vi "rm.server.visualize.vi"(8 "error in (no error)":errorcluster, 11 "Item Ref in":T1 format="%.0x") -> (0 "error out":errorcluster, 3 "Item Ref out":T1 format="%.0x")   [LabVIEW 2016, in "RM.Server.lvlib"]
uses:
  RM.Server.lvlib
  <vilib>/NI Veristand/Custom Device API/Custom Device Item Ref.ctl
  viz_entry.ctl
  viz_type.ctl
  viz_show.ctl
  viz_state.ctl
  <vilib>/NI Veristand/Custom Device Tools/Custom Device Utility Library/Custom Device Utility Library.lvlib
  <vilib>/NI Veristand/Custom Device API/Custom Device API.lvlib
panel:
  in  "Collapse Sidebar":bool
  in  "Collapse Sort Options":bool
  in  "Sort By...":T2 items=["RIO device", "resource", "input type", "datatype", "reserver"]
  in  "Collapse Filter Options":bool
  in  "Show":T3
  in  "Display":i32(listbox)
  out "selected values":bool[](array[boolean])
  in  "table":i32(listbox)
  out "resource entries":T4[](array[typedef]) {"FPGA CD Ref" format="%.0x"; "reserver" format="%.0x"}
  # "Options"
  # "Sort"
  # "Filter"
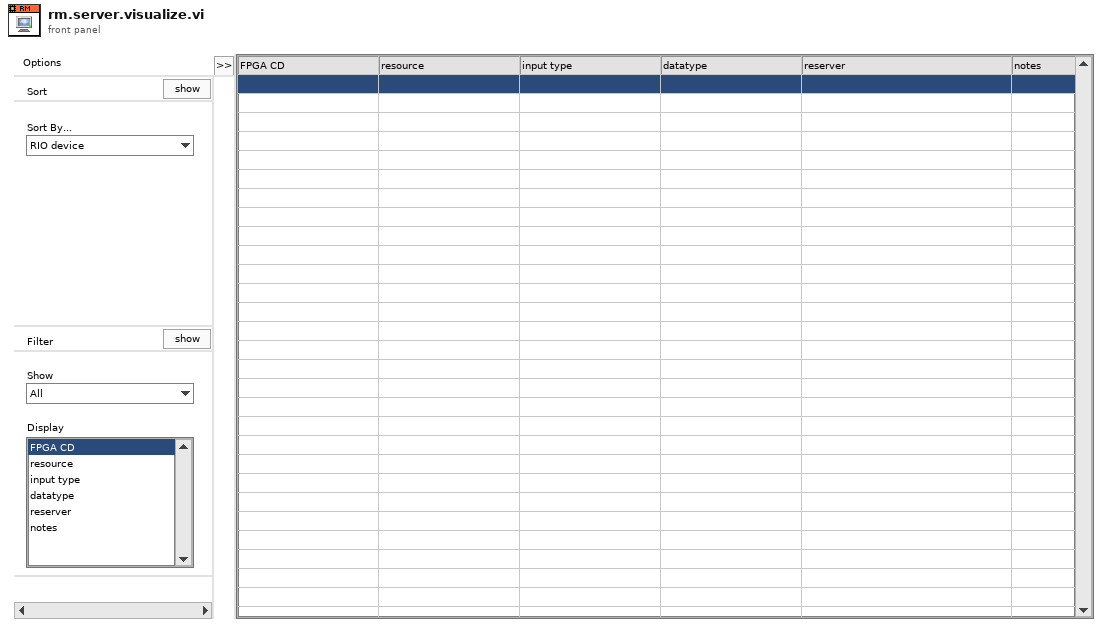
[diagram p1: front panel]
types:
  T1 = typedef "Custom Device API.lvlib/Custom Device Item Ref.ctl" = u64
  T2 = typedef "RM.Server.lvlib/viz_type.ctl" = u16
  T3 = typedef "RM.Server.lvlib/viz_show.ctl" = enum16{"All", "Mapped", "Unmapped"}
  T4 = typedef "RM.Server.lvlib/viz_entry.ctl" = cluster{"FPGA CD Ref":T1, "resource name":string, "input type":string, "datatype":string, "reserver":T1, "notes":string}
  T5 = typedef "RM.Server.lvlib/viz_state.ctl" = enum16{"shutdown"}
  T6 = typedef "RM.Server.lvlib/viz_command.ctl" = cluster{"state":T5, "data":variant}
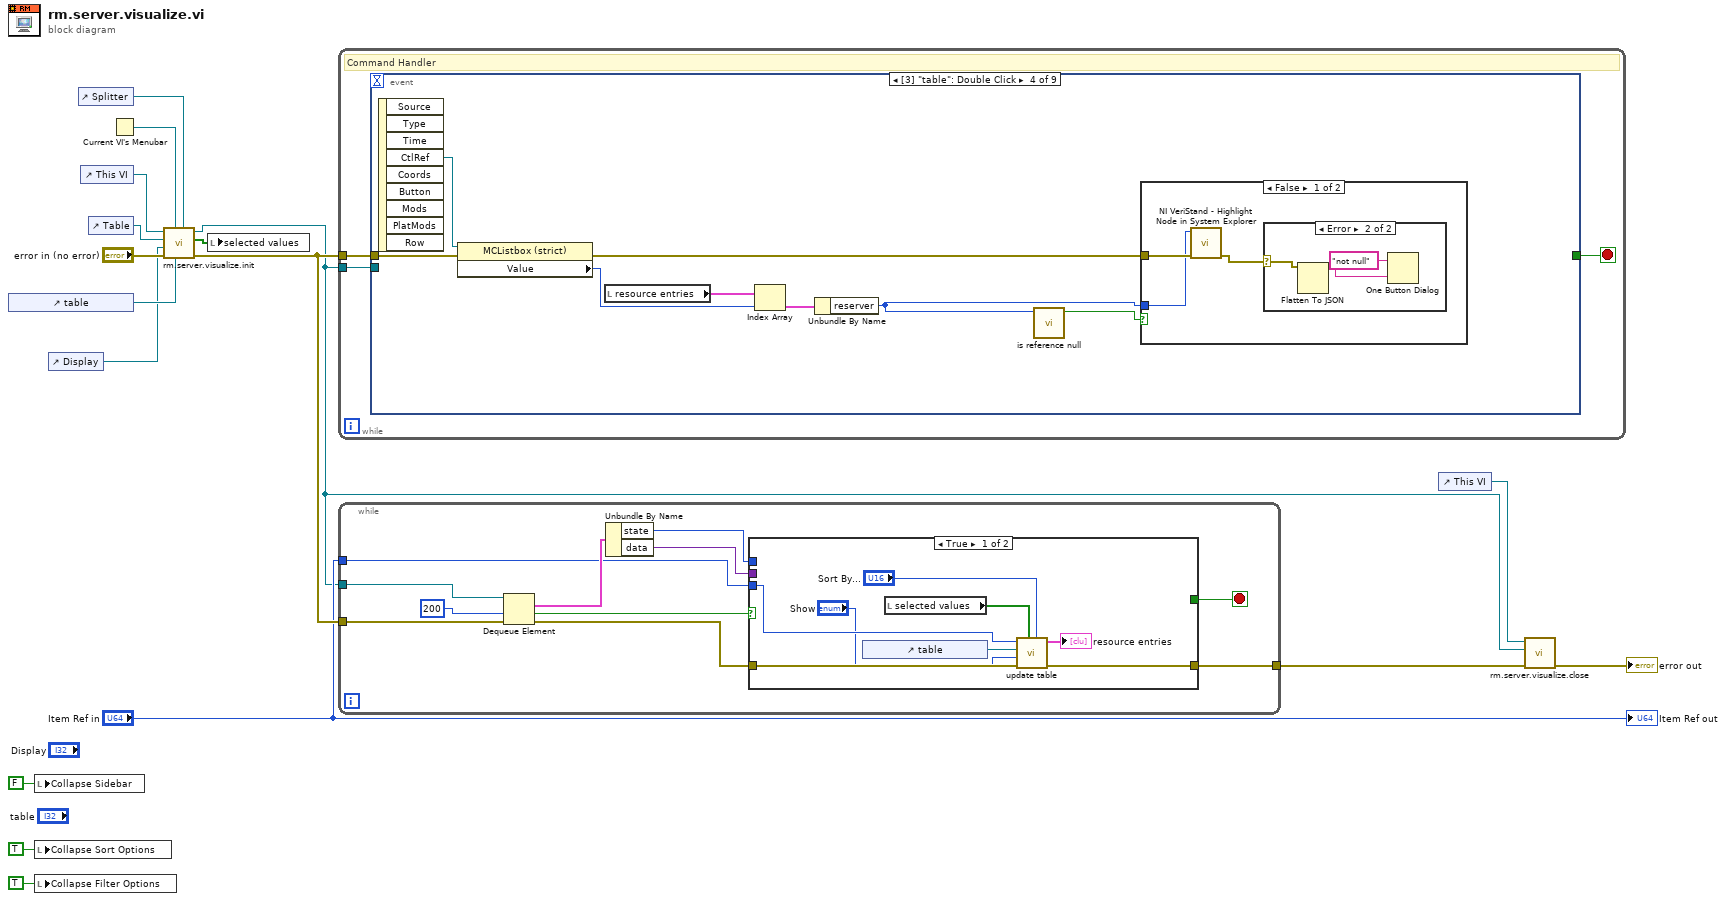
[diagram p0: block diagram]
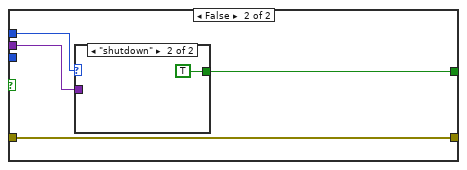
[diagram p2: hidden frame]
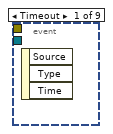
[diagram p4: hidden frame]
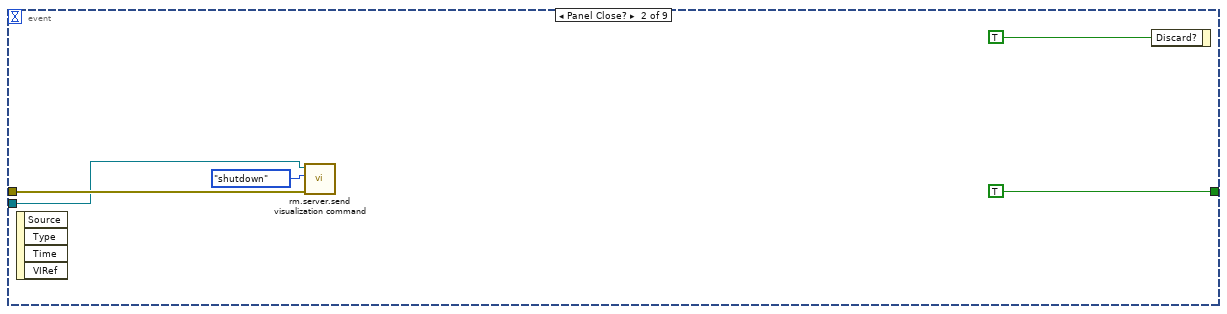
[diagram p5: hidden frame]
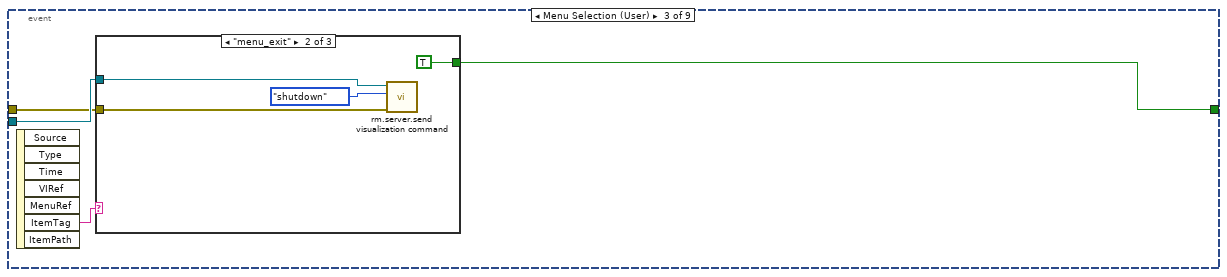
[diagram p6: hidden frame]
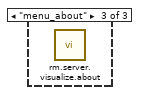
[diagram p8: hidden frame]
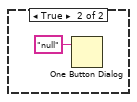
[diagram p10: hidden frame]
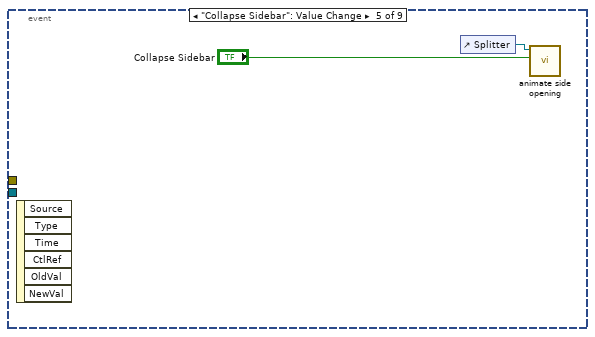
[diagram p11: hidden frame]
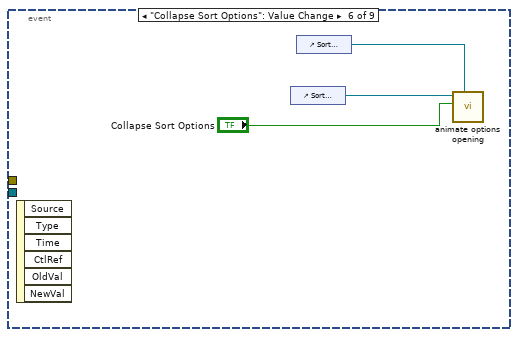
[diagram p12: hidden frame]
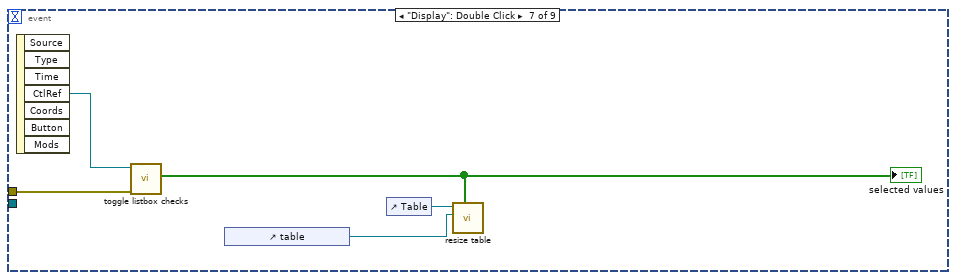
[diagram p13: hidden frame]
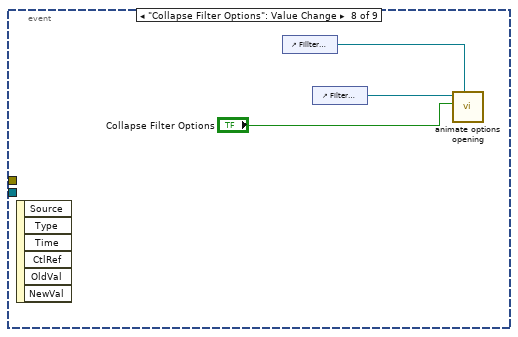
[diagram p14: hidden frame]
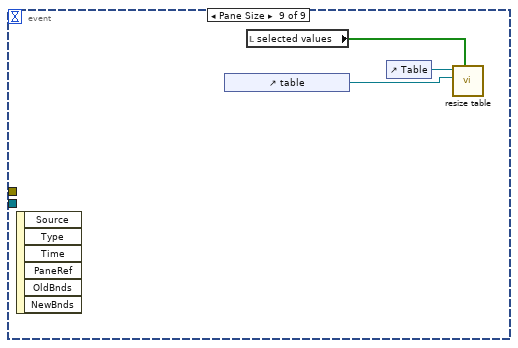
[diagram p15: hidden frame]
diagram:
  n1 = control-ref of="table"() -> (w4:refnum<vi>)
  n2 = local write "Collapse Sidebar"(FALSE ("Collapse Sidebar")) -> ()
  n3 = local write "Collapse Sort Options"(TRUE ("Collapse Sort Options")) -> ()
  n4 = local write "Collapse Filter Options"(TRUE ("Collapse Sort Options")) -> ()
  n5 = control-ref of="Display"() -> (w1:refnum<vi>)
  n6 = control-ref of="Splitter"() -> (w8:refnum<vi>)
  n7 = control-ref of="This VI"() -> (w14:refnum<vi>)
  n8 = control-ref of="Table"() -> (w3:refnum<vi>)
  n9 = Current VI's Menubar() -> (w9:refnum<k9>)
  n10 = call "rm.server.visualize.init.vi"("Splitter"=w8, "MCLB Reference"=w4, "menu reference in"=w9, "error in (no error)"="error in (no error)", "display"=w1, "Table Pane in"=w3, "VI in"=w14) -> ("error out"=w16:errorcluster, "selected values"=w2:bool[], "Queue out"=w10:refnum<queue>)  [unwired: 2 in]
  n11 = local write "selected values"(w2) -> ()
  n12 = while {
    tunnel: w10 -> [w19]
    tunnel: w16 -> [w18]
    stop <- w20 stop-if-true
    # "Command Handler"
    n13 = event shown="[3] \"table\": Double Click" {
      selector: _ -> [_ _ _ _ _ _ _ _ _]
      dyn-events: _ -> [_ _ _ _ _ _ _ _ _]
      timeout: _ -> [_ _ _ _ _ _ _ _ _]
      tunnel: [_ TRUE w28 _ _ _ _ _ _] -> w20
      tunnel: w19 -> [_ w21 w27 _ _ _ _ _ _]
      tunnel: w18 -> [_ w22 w26 w40 _ _ w57 _ _]
      event Timeout {
        n14 = event-data() -> ()  [unwired: 1 in, 3 out]
      }
      event Panel Close? {
        n15 = event-data() -> ()  [unwired: 1 in, 4 out]
        n16 = call "rm.server.send visualization command.vi"("error in (no error)"=w22, "state"=viz_state."shutdown" ("viz_state"), "Queue in"=w21) -> ()  [unwired: 8 in, 1 out]
        n17 = event-data("Discard?"=TRUE ("SilentShutdown")) -> ()  [unwired: 1 in, 1 out]
      }
      event Menu Selection (User) {
        n18 = event-data() -> ("ItemTag"=w29:string)  [unwired: 1 in, 6 out]
        n19 = case shown="\"menu_exit\"" w29 {
          tunnel: [_ TRUE _] -> w28
          tunnel: w27 -> [_ w32 _]
          tunnel: w26 -> [_ w30 _]
          frame Default {
          }
          frame "menu_exit" {
            n20 = call "rm.server.send visualization command.vi"("error in (no error)"=w30, "state"=viz_state."shutdown" ("viz_state"), "Queue in"=w32) -> ()  [unwired: 8 in, 1 out]
          }
          frame "menu_about" {
            n21 = call "rm.server.visualize.about.vi"() -> ()  [unwired: 12 in]
          }
        }
      }
      event "table": Double Click {
        n22 = event-data() -> ("CtlRef"=w41:refnum<vi>)  [unwired: 1 in, 8 out]
        n23 = property class="MCListbox (strict)"(reference=w41, error in=w40) -> (error out=w38:errorcluster, "Value"=w39:i32)  [unwired: 1 out]
        n24 = local read "resource entries"() -> (w37:T4[])
        n25 = Index Array(array=w37, index=w39) -> (element=w36:T4)
        n26 = Unbundle By Name(w36) -> ("reserver"=w35:T1)
        n27 = call "is reference null.vi"("reserver"=w35) -> ("Boolean"=w34:bool)  [unwired: 10 in]
        n28 = case shown="False" w34 {
          tunnel: w38 -> [w44 _]
          tunnel: w35 -> [w43 _]
          frame False {
            n29 = call <vilib>:"NI VeriStand - Highlight Node in System Explorer.vi"("error in (no error)"=w44, "Item Ref in"=w43) -> ("error out"=w42:errorcluster)  [unwired: 8 in, 1 out]
            n30 = case shown="Error" w42 {
              selector: w42 -> [_ w46]
              frame No Error {
              }
              frame Error {
                n31 = Flatten To JSON(anything=w46) -> (JSON string=w45:string)  [unwired: 2 in, 1 out]
                n32 = One Button Dialog(message="not null", button name ("OK")=w45) -> ()  [unwired: 1 out]
              }
            }
          }
          frame True {
            n33 = One Button Dialog(message="null") -> ()  [unwired: 1 in, 1 out]
          }
        }
      }
      event "Collapse Sidebar": Value Change {
        n34 = event-data() -> ()  [unwired: 1 in, 6 out]
        n35 = control-ref of="Splitter"() -> (w50:refnum<vi>)
        n36 = call "animate side opening.vi"("expand/collapse"="Collapse Sidebar", "Splitter in"=w50) -> ()  [unwired: 10 in]
      }
      event "Collapse Sort Options": Value Change {
        n37 = event-data() -> ()  [unwired: 1 in, 6 out]
        n38 = control-ref of="Sort Options-Filter Header"() -> (w52:refnum<vi>)
        n39 = control-ref of="Sort Header-Sort Options"() -> (w51:refnum<vi>)
        n40 = call "animate options opening.vi"("Top Splitter in"=w51, "expand/collapse"="Collapse Sort Options", "Bottom Splitter in"=w52) -> ()  [unwired: 9 in]
      }
      event "Display": Double Click {
        n41 = event-data() -> ("CtlRef"=w58:refnum<vi>)  [unwired: 1 in, 6 out]
        n42 = call "toggle listbox checks.vi"("error in (no error)"=w57, "ListBox in"=w58) -> ("selected values"=w54:bool[])  [unwired: 8 in, 1 out]
        "selected values" <- w54
        n43 = control-ref of="table"() -> (w55:refnum<vi>)
        n44 = control-ref of="Table"() -> (w56:refnum<vi>)
        n45 = call "resize table.vi"("selected values"=w54, "table"=w55, "Pane in"=w56) -> ()  [unwired: 8 in, 1 out]
      }
      event "Collapse Filter Options": Value Change {
        n46 = event-data() -> ()  [unwired: 1 in, 6 out]
        n47 = control-ref of="Fillter Header-Filter Options"() -> (w60:refnum<vi>)
        n48 = control-ref of="Filter Options-Bottom"() -> (w61:refnum<vi>)
        n49 = call "animate options opening.vi"("Top Splitter in"=w60, "expand/collapse"="Collapse Filter Options", "Bottom Splitter in"=w61) -> ()  [unwired: 9 in]
      }
      event Pane Size {
        n50 = event-data() -> ()  [unwired: 1 in, 6 out]
        n51 = control-ref of="table"() -> (w63:refnum<vi>)
        n52 = local read "selected values"() -> (w62:bool[])
        n53 = control-ref of="Table"() -> (w64:refnum<vi>)
        n54 = call "resize table.vi"("selected values"=w62, "table"=w63, "Pane in"=w64) -> ()  [unwired: 8 in, 1 out]
      }
    }
  }
  n55 = while {
    tunnel: w10 -> [w75]
    tunnel: w16 -> [w72]
    tunnel: "Item Ref in" -> [w70]
    tunnel: [w69] -> w13
    stop <- w73 stop-if-true
    n56 = Dequeue Element(queue=w75, timeout in ms (-1)=200, error in (no error)=w72) -> (element=w74:T6, timed out?=w67:bool, error out=w71:errorcluster)  [unwired: 1 out]
    n57 = Unbundle By Name(w74) -> ("state"=w66:T5, "data"=w65:variant)
    n58 = case shown="True" w67 {
      tunnel: [_ w87] -> w73
      tunnel: w71 -> [w83 w86]
      tunnel: w70 -> [w79 _]
      tunnel: [w82 w86] -> w69
      tunnel: w66 -> [_ w85]
      tunnel: w65 -> [_ w84]
      frame True {
        n59 = control-ref of="table"() -> (w80:refnum<vi>)
        n60 = local read "selected values"() -> (w78:bool[])
        n61 = call "update table.vi"("Sort By..."="Sort By...", "selected values"=w78, "error in (no error)"=w83, "Show"="Show", "MulticolumnListbox in"=w80, "Item Ref in"=w79) -> ("error out"=w82:errorcluster, "resource entries"=→"resource entries":T4[])  [unwired: 4 in]
      }
      frame False {
        n62 = case shown="\"shutdown\"" w85 {
          tunnel: [_ TRUE] -> w87
          tunnel: w84 -> [_ _]
          frame Default {
          }
          frame "shutdown" {
          }
        }
      }
    }
  }
  n63 = control-ref of="This VI"() -> (w11:refnum<vi>)
  n64 = call "rm.server.visualize.close.vi"("error in (no error)"=w13, "Queue in"=w10, "reference"=w11) -> ("error out"=→"error out":errorcluster)  [unwired: 8 in]
  "Item Ref out" <- "Item Ref in"
